vi "ConfigurationPulse.vi"() -> ()   [LabVIEW 2022 SP3]
uses:
  <vilib>/regexp/Match Regular Expression.xnode
panel:
  in  "Tab Control":T1(tab)
  out "COM Port Found":bool
  out "Detected COM Port":string
  in  "Start Search":bool
  in  "Set High1 Duration Time":bool
  in  "High1 Time (1-255)":i16=1 min=1 max=255 step=1
  out "High1 Duration in nsec":dbl
  out "High1 Sent":bool
  in  "Set Low1 Duration Time":bool
  in  "Low1 Time (1-255)":i16=1 min=1 max=255 step=1
  out "Low1 Duration in nsec":dbl
  out "Low1 Sent":bool
  in  "Set High2 Duration Time":bool
  in  "High2 Time (1-255)":i16=1 min=1 max=255 step=1
  out "High2 Duration in nsec":dbl
  out "High2 Sent":bool
  out "Duration of 2nd Pulse":dbl
  out "Duration of Dead Time":dbl
  out "Duration of 1st Pulse":dbl
  out "String":string
  out "Pulse Sent":bool
  in  "Send Pulse":bool
  in  "Try from the beginning":bool
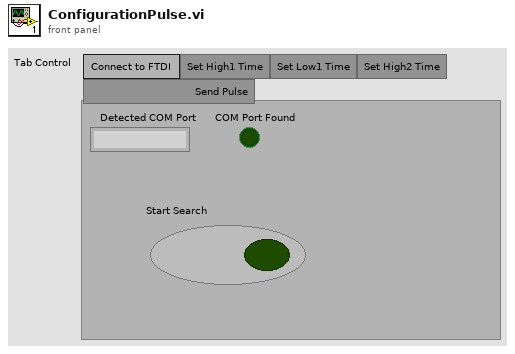
[diagram p1: front panel]
types:
  T1 = enum32{"Connect to FTDI ", "Set High1 Time", "Set Low1 Time", "Set High2 Time", "                                   Send Pulse"}
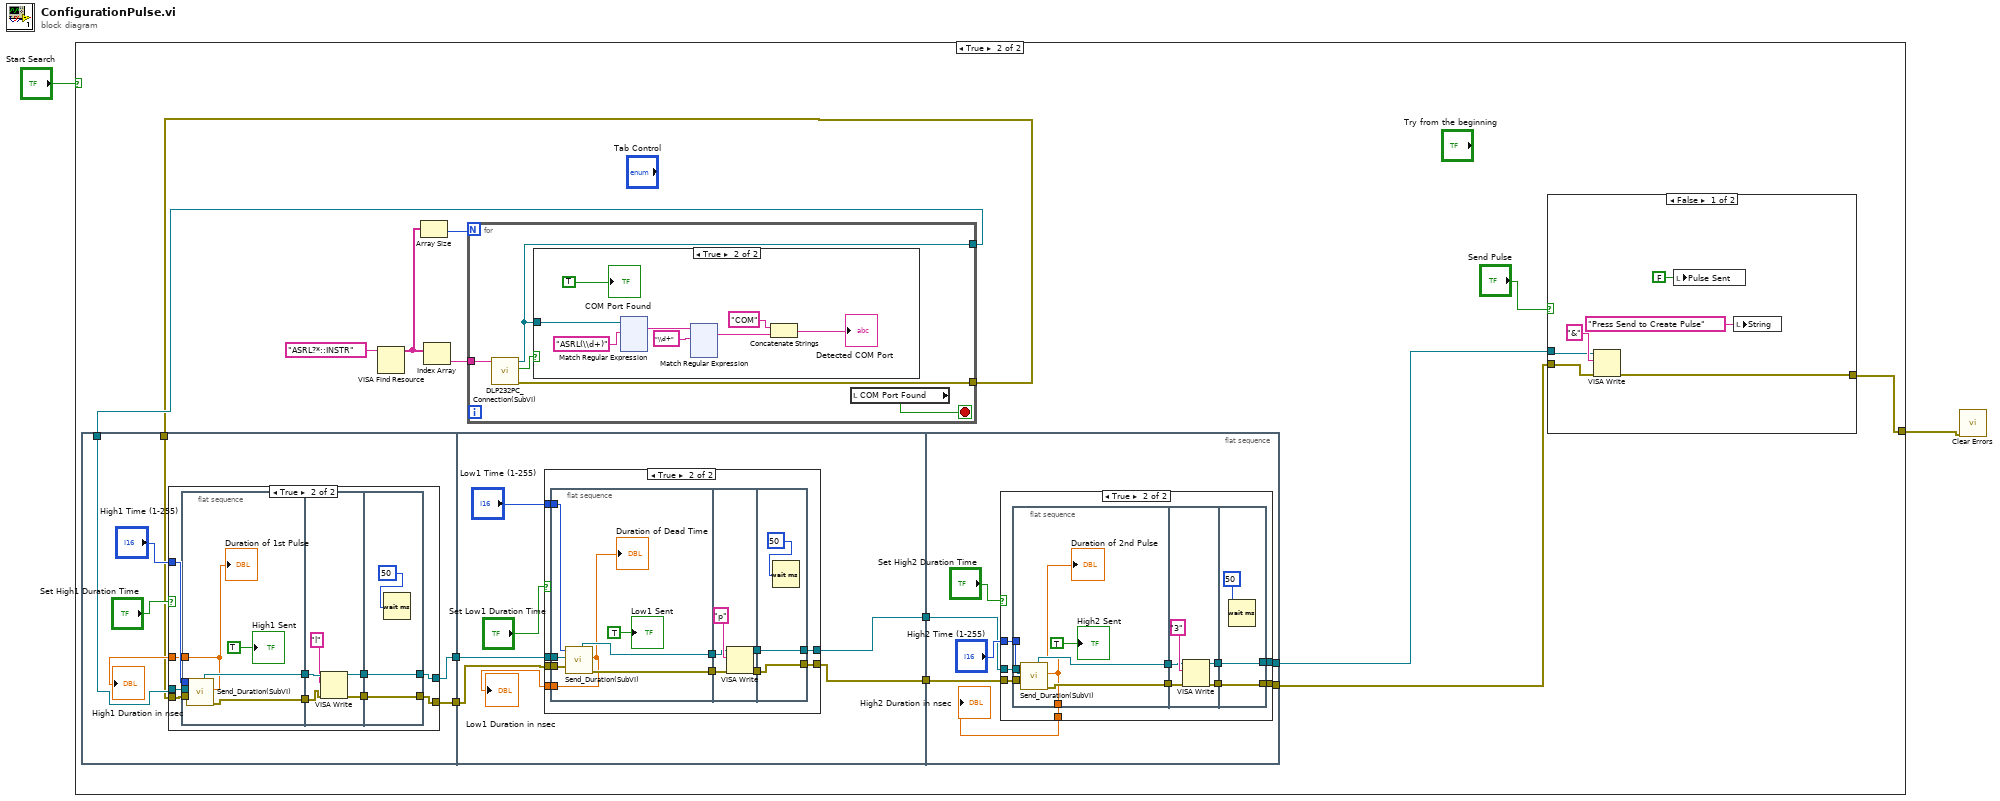
[diagram p0: block diagram]
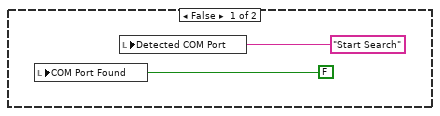
[diagram p2: hidden frame]
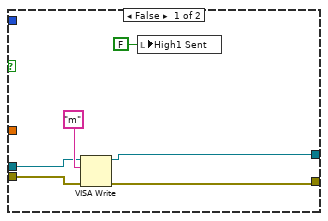
[diagram p3: hidden frame]
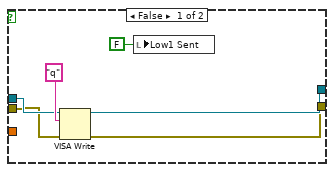
[diagram p4: hidden frame]
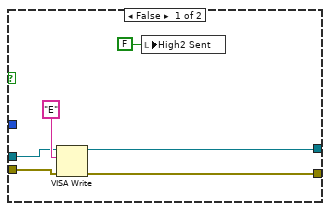
[diagram p5: hidden frame]
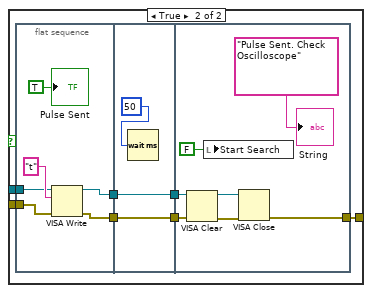
[diagram p6: hidden frame]
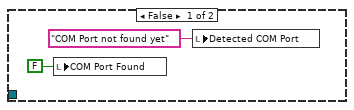
[diagram p7: hidden frame]
diagram:
  n1 = case shown="True" "Start Search" {
    tunnel: [_ w13] -> w1
    frame False {
      n2 = local write "COM Port Found"(FALSE ("Send Pulse")) -> ()
      n3 = local write "Detected COM Port"("Start Search" ("Detected COM Port")) -> ()
    }
    frame True {
      n4 = flat-sequence {
        tunnel: [w22] -> w12
        tunnel: [w21] -> w11
        tunnel: w6 -> [w20]
        tunnel: w5 -> [w19]
        tunnel: w12 -> [w59]
        tunnel: w11 -> [w58]
        tunnel: [w57] -> w8
        tunnel: [w56] -> w7
        tunnel: [w97] -> w10
        tunnel: [w96] -> w9
        tunnel: w8 -> [w95]
        tunnel: w7 -> [w94]
        frame #0 {
          n5 = case shown="True" "Set High1 Duration Time" {
            tunnel: w20 -> [w30 w37]
            tunnel: w19 -> [w29 w36]
            tunnel: "High1 Time (1-255)" -> [_ w35]
            tunnel: [_ w34] -> w25
            tunnel: [w27 w33] -> w22
            tunnel: [w26 w32] -> w21
            frame False {
              n6 = VISA Write(VISA resource name=w30, write buffer="m", error in (no error)=w29) -> (VISA resource name out=w27:refnum<visa-resource-name>, error out=w26:errorcluster)  [unwired: 1 out]
              n7 = local write "High1 Sent"(FALSE ("High1 Sent")) -> ()
            }
            frame True {
              n8 = flat-sequence {
                tunnel: w37 -> [w47]
                tunnel: w36 -> [w46]
                tunnel: [w45] -> w41
                tunnel: [w44] -> w40
                tunnel: w35 -> [w43]
                tunnel: [w42] -> w34
                tunnel: w41 -> [w52]
                tunnel: [w52] -> w39
                tunnel: w40 -> [w50]
                tunnel: [w49] -> w38
                tunnel: w39 -> [w54]
                tunnel: w38 -> [w53]
                tunnel: [w54] -> w33
                tunnel: [w53] -> w32
                frame #0 {
                  n9 = call "Send_Duration(SubVI).vi"("error in (no error)"=w46, "VISA resource name"=w47, "Set High1 Time"=w43) -> ("error out"=w44:errorcluster, "High1 Time(ns)"=w42:dbl, "VISA resource name out"=w45:refnum<visa-resource-name>)  [unwired: 3 in, 3 out]
                  "Duration of 1st Pulse" <- w42
                  "High1 Sent" <- TRUE ("High1 Sent")
                }
                frame #1 {
                  n10 = VISA Write(VISA resource name=w52, write buffer="l", error in (no error)=w50) -> (error out=w49:errorcluster)  [unwired: 2 out]
                }
                frame #2 {
                  n11 = Wait (ms)(milliseconds to wait=u32 50) -> ()  [unwired: 1 out]
                }
              }
            }
          }
          "High1 Duration in nsec" <- w25
        }
        frame #1 {
          n12 = case shown="True" "Set Low1 Duration Time" {
            tunnel: w58 -> [w66 w73]
            tunnel: w59 -> [w67 w74]
            tunnel: [_ w72] -> w60
            tunnel: [w64 w71] -> w57
            tunnel: [w63 w70] -> w56
            tunnel: "Low1 Time (1-255)" -> [_ w69]
            frame False {
              n13 = VISA Write(VISA resource name=w67, write buffer="q", error in (no error)=w66) -> (VISA resource name out=w64:refnum<visa-resource-name>, error out=w63:errorcluster)  [unwired: 1 out]
              n14 = local write "Low1 Sent"(FALSE ("Low1 Sent")) -> ()
            }
            frame True {
              n15 = flat-sequence {
                tunnel: w74 -> [w84]
                tunnel: [w83] -> w78
                tunnel: [w82] -> w77
                tunnel: w73 -> [w81]
                tunnel: [w79] -> w72
                tunnel: w69 -> [w80]
                tunnel: w78 -> [w89]
                tunnel: w77 -> [w88]
                tunnel: [w87] -> w76
                tunnel: [w86] -> w75
                tunnel: [w92] -> w71
                tunnel: w76 -> [w92]
                tunnel: w75 -> [w91]
                tunnel: [w91] -> w70
                frame #0 {
                  n16 = call "Send_Duration(SubVI).vi"("error in (no error)"=w81, "VISA resource name"=w84, "Set High1 Time"=w80) -> ("error out"=w82:errorcluster, "High1 Time(ns)"=w79:dbl, "VISA resource name out"=w83:refnum<visa-resource-name>)  [unwired: 3 in, 3 out]
                  "Duration of Dead Time" <- w79
                  "Low1 Sent" <- TRUE ("Low1 Sent")
                }
                frame #1 {
                  n17 = VISA Write(VISA resource name=w89, write buffer="p", error in (no error)=w88) -> (VISA resource name out=w87:refnum<visa-resource-name>, error out=w86:errorcluster)  [unwired: 1 out]
                }
                frame #2 {
                  n18 = Wait (ms)(milliseconds to wait=u32 50) -> ()  [unwired: 1 out]
                }
              }
            }
          }
          "Low1 Duration in nsec" <- w60
        }
        frame #2 {
          n19 = case shown="True" "Set High2 Duration Time" {
            tunnel: w94 -> [w104 w112]
            tunnel: w95 -> [w105 w111]
            tunnel: [w102 w110] -> w97
            tunnel: [w101 w109] -> w96
            tunnel: "High2 Time (1-255)" -> [_ w108]
            tunnel: [_ w107] -> w100
            frame False {
              n20 = VISA Write(VISA resource name=w105, write buffer="E", error in (no error)=w104) -> (VISA resource name out=w102:refnum<visa-resource-name>, error out=w101:errorcluster)  [unwired: 1 out]
              n21 = local write "High2 Sent"(FALSE ("High2 Sent")) -> ()
            }
            frame True {
              n22 = flat-sequence {
                tunnel: w111 -> [w123]
                tunnel: [w121] -> w116
                tunnel: [w120] -> w115
                tunnel: w112 -> [w119]
                tunnel: w108 -> [w118]
                tunnel: [w117] -> w107
                tunnel: w116 -> [w127]
                tunnel: w115 -> [w126]
                tunnel: [w125] -> w114
                tunnel: [w124] -> w113
                tunnel: [w131] -> w110
                tunnel: w114 -> [w131]
                tunnel: [w130] -> w109
                tunnel: w113 -> [w130]
                frame #0 {
                  n23 = call "Send_Duration(SubVI).vi"("error in (no error)"=w119, "VISA resource name"=w123, "Set High1 Time"=w118) -> ("error out"=w120:errorcluster, "High1 Time(ns)"=w117:dbl, "VISA resource name out"=w121:refnum<visa-resource-name>)  [unwired: 3 in, 3 out]
                  "Duration of 2nd Pulse" <- w117
                  "High2 Sent" <- TRUE ("High2 Sent")
                }
                frame #1 {
                  n24 = VISA Write(VISA resource name=w127, write buffer="3", error in (no error)=w126) -> (VISA resource name out=w125:refnum<visa-resource-name>, error out=w124:errorcluster)  [unwired: 1 out]
                }
                frame #2 {
                  n25 = Wait (ms)(milliseconds to wait=u32 50) -> ()  [unwired: 1 out]
                }
              }
            }
          }
          "High2 Duration in nsec" <- w100
        }
      }
      n26 = VISA Find Resource(11:"ASRL?*::INSTR" ("expression (\"?*\")")) -> (3:w16:string[])  [unwired: 2 in, 2 out]
      n27 = Array Size(array=w16) -> (size(s)=w18:i32)
      n28 = Index Array(array=w16) -> (element=w17:string)  [unwired: 1 in]
      n29 = for {
        N: w18 -> [_]
        tunnel: w17 -> [w165]
        tunnel: [w162] -> w6
        tunnel: [w161] -> w5
        stop <- w163 stop-if-true
        n30 = call "DLP232PC_Connection(SubVI).vi"("String"=w165) -> ("error out"=w161:errorcluster, "Boolean"=w164:bool, "VISA Refnum out"=w162:refnum<visa-resource-name>)  [unwired: 8 in]
        n31 = case shown="True" w164 {
          tunnel: w162 -> [_ w168]
          frame False {
            n32 = local write "COM Port Found"(FALSE ("COM Port Found")) -> ()
            n33 = local write "Detected COM Port"("COM Port not found yet" ("Detected COM Port")) -> ()
          }
          frame True {
            n34 = xnode "Match Regular Expression"("input string"=w168, "regular expression"="ASRL(\\d+)") -> ("whole match"=w172:string)  [unwired: 4 in, 4 out]
            n35 = xnode "Match Regular Expression"("input string"=w172, "regular expression"="\\d+") -> ("whole match"=w170:string)  [unwired: 4 in, 4 out]
            n36 = Concatenate Strings("COM" ("string"), w170) -> (→"Detected COM Port":string)
            "COM Port Found" <- TRUE ("DLP-232PC Found")
          }
        }
        n37 = local read "COM Port Found"() -> (w163:bool)
      }
      n38 = case shown="False" "Send Pulse" {
        tunnel: w10 -> [w136 w144]
        tunnel: w9 -> [w135 w143]
        tunnel: [w134 w138] -> w13
        frame False {
          n39 = VISA Write(VISA resource name=w136, write buffer="&", error in (no error)=w135) -> (error out=w134:errorcluster)  [unwired: 2 out]
          n40 = local write "Pulse Sent"(FALSE ("Pulse Sent")) -> ()
          n41 = local write "String"("Press Send to Create Pulse" ("String")) -> ()
        }
        frame True {
          n42 = flat-sequence {
            tunnel: w144 -> [w149]
            tunnel: w143 -> [w148]
            tunnel: [w146] -> w142
            tunnel: [w145] -> w139
            tunnel: w142 -> [w152]
            tunnel: [w152] -> w141
            tunnel: [w151] -> w140
            tunnel: w139 -> [w151]
            tunnel: w141 -> [w157]
            tunnel: w140 -> [w156]
            tunnel: [w155] -> w138
            frame #0 {
              n43 = VISA Write(VISA resource name=w149, write buffer="t", error in (no error)=w148) -> (VISA resource name out=w146:refnum<visa-resource-name>, error out=w145:errorcluster)  [unwired: 1 out]
              "Pulse Sent" <- TRUE ("Pulse Sent")
            }
            frame #1 {
              n44 = Wait (ms)(milliseconds to wait=u32 50) -> ()  [unwired: 1 out]
            }
            frame #2 {
              n45 = VISA Clear(VISA resource name=w157, error in (no error)=w156) -> (VISA resource name out=w158:refnum<visa-resource-name>, error out=w159:errorcluster)
              n46 = local write "Start Search"(FALSE ("Start Search")) -> ()
              n47 = VISA Close(VISA resource name=w158, error in (no error)=w159) -> (error out=w155:errorcluster)
              "String" <- "Pulse Sent. Check Oscilloscope" ("String")
            }
          }
        }
      }
    }
  }
  n48 = call <vilib>:"Clear Errors.vi"("error in (no error)"=w1) -> ()  [unwired: 5 in, 2 out]
